vi "Prepare Config.vi"(8 "Error In":errorcluster, 11 "IConfigIn":refnum<class "IConfig.lvclass">) -> (0 "Error Out":errorcluster, 3 "IConfigOut":refnum<class "IConfig.lvclass">)   [LabVIEW 2019, in "IConfig.lvclass"]
uses:
  IConfig.lvclass
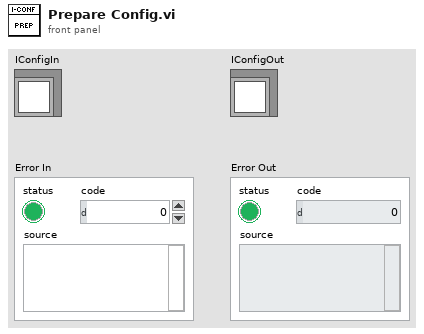
[diagram p1: front panel]
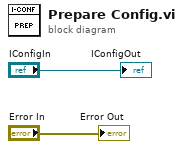
[diagram p0: block diagram]
diagram:
  "IConfigOut" <- "IConfigIn"
  "Error Out" <- "Error In"
